vi "Set Perimiters_B.vi"(11 "Plant Regions in":map{T1, bool[]}[](array[numeric])) -> (3 "Plant Regions out":map{T1, bool[]}[](array[numeric]))   [LabVIEW 2024]
uses:
  Utility/Universal Utility/TypeDefs_Utility/Cluster_Row-Column.ctl
  Utility/Universal Utility/TypeDefs_Utility/ENUM_4 Directions U-D-L-R.ctl
  <vilib>/Utility/miscctls.llb/LVMapReplaceAction.ctl
  9ec40043-fd1c-4aa8-aa2f-c598280360ae.vi
  9ec40043-fd1c-4aa8-aa2f-c598280360ae.vi/0a5f5d0f-6921-449f-9499-5f6c7f3eae0e.vi
  9ec40043-fd1c-4aa8-aa2f-c598280360ae.vi/2f57c213-34d0-4fb8-93c4-9da21d141025.vi
  <vilib>/Utility/error.llb/Trim Whitespace.vi
  <vilib>/Utility/error.llb/Trim Whitespace One-Sided.vi
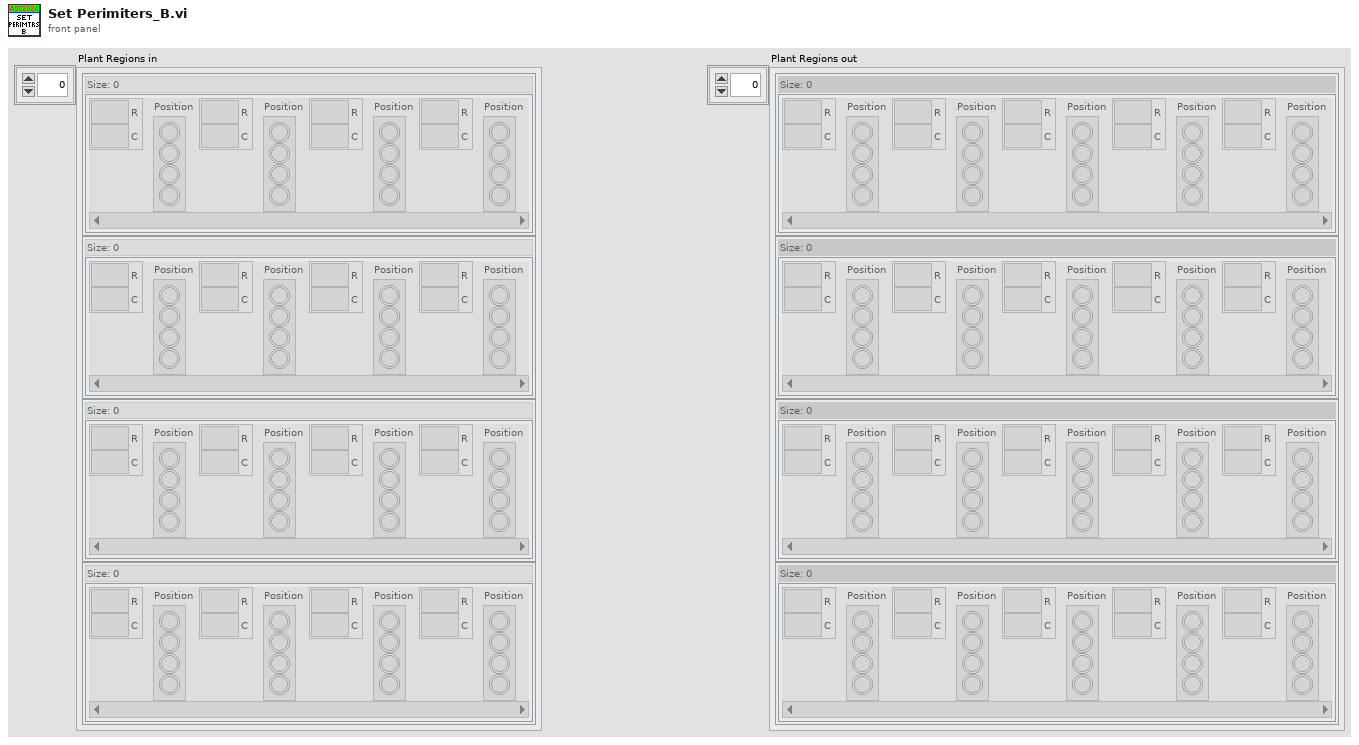
[diagram p1: front panel]
types:
  T1 = typedef "Cluster_Row-Column.ctl" = cluster{"R":i32, "C":i32}
  T2 = typedef "ENUM_4 Directions U-D-L-R.ctl" = enum16{"Up;-1,0", "Right;0,1", "Down;1,0", "Left;0,-1"}
  T3 = typedef "LVMapReplaceAction.ctl" = enum32{"Modify Entry only if found", "Add or Modify Entry", "Delete Entry"}
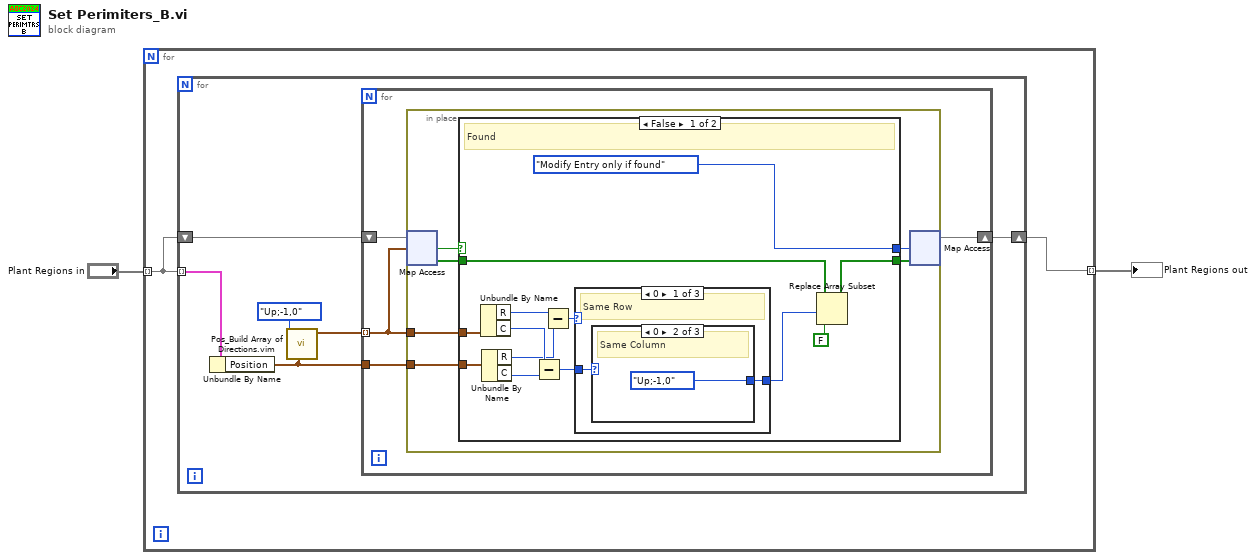
[diagram p0: block diagram]
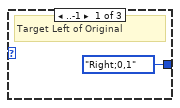
[diagram p2: hidden frame]
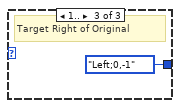
[diagram p3: hidden frame]
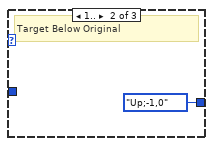
[diagram p4: hidden frame]
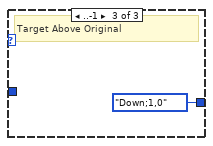
[diagram p5: hidden frame]
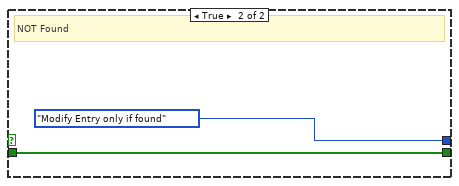
[diagram p6: hidden frame]
diagram:
  n1 = for {
    tunnel: "Plant Regions in" -> [w4] mode=indexing
    tunnel: [w3] -> w1 mode=indexing
    n2 = for {
      tunnel: w4 -> [w10] mode=indexing
      shift-right: [w7] -> w3
      shift-left: w4 -> [w8]
      n3 = Unbundle By Name(w10) -> ("Position"=w5:T1)
      n4 = call "Pos_Build Array of Directions.vim"("Positon"=w5, "Direction"=ENUM_4_Directions_U-D-L-R."Up;-1,0") -> ("Direction Positions Out"=w6:T1[])  [unwired: 9 in]
      n5 = for {
        tunnel: w6 -> [w12] mode=indexing
        shift-right: [w13] -> w7
        shift-left: w8 -> [w14]
        tunnel: w5 -> [w11]
        n6 = in-place {
          in-place-border: w12 -> [w16]
          in-place-border: w11 -> [w15]
          n7 = in-place-map #1(w14, w12) -> (w20:bool[], w18:bool)  [unwired: 1 in]
          n8 = case shown="False" w18 {
            tunnel: w20 -> [w23 w41]
            tunnel: [LVMapReplaceAction."Modify Entry only if found" ("action") LVMapReplaceAction."Modify Entry only if found" ("action")] -> w19
            tunnel: [w24 w41] -> w17
            tunnel: w16 -> [w32 _]
            tunnel: w15 -> [w31 _]
            frame False {
              # "Found"
              n9 = Unbundle By Name(w32) -> ("R"=w28:i32, "C"=w29:i32)
              n10 = Unbundle By Name(w31) -> ("R"=w27:i32, "C"=w30:i32)
              n11 = Subtract(x=w29, y=w30) -> (x-y=w25:i32)
              n12 = Subtract(x=w28, y=w27) -> (x-y=w26:i32)
              n13 = case shown="0" w26 {
                tunnel: w25 -> [w35 _ _]
                tunnel: [w34 ENUM_4_Directions_U-D-L-R."Up;-1,0" ("Direction") ENUM_4_Directions_U-D-L-R."Down;1,0" ("Direction")] -> w22
                frame 0 {
                  # "Same Row"
                  n14 = case shown="0" w35 {
                    tunnel: [ENUM_4_Directions_U-D-L-R."Right;0,1" ("Direction") ENUM_4_Directions_U-D-L-R."Up;-1,0" ("Direction") ENUM_4_Directions_U-D-L-R."Left;0,-1" ("Direction")] -> w34
                    frame ..-1 {
                      # "Target Left of Original"
                    }
                    frame 0 {
                      # "Same Column"
                    }
                    frame 1.. {
                      # "Target Right of Original"
                    }
                  }
                }
                frame 1.. {
                  # "Target Below Original"
                }
                frame ..-1 {
                  # "Target Above Original"
                }
              }
              n15 = Replace Array Subset(array=w23, new element=FALSE, index=w22) -> (w24:bool[])
            }
            frame True {
              # "NOT Found"
            }
          }
          n16 = in-place-map #1(w17, w19) -> (w13:map{T1, bool[]})  [unwired: 2 out]
        }
      }
    }
  }
  "Plant Regions out" <- w1
